vi "Init.vi"(10 "String Indicator":string) -> (3 "String Indicator Msg Strategy out":refnum<class "String Indicator Msg Strategy.lvclass">)   [LabVIEW 2021, in "jettl Msg String Indicator.lvlib" / "String Indicator Msg Strategy.lvclass"]
uses:
  String Indicator Msg Strategy.lvclass
  String Indicator Msg Strategy.lvclass/String Indicator Msg Strategy.ctl
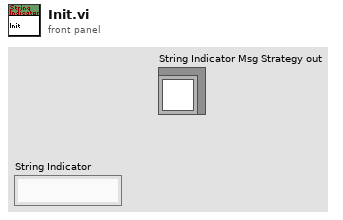
[diagram p1: front panel]
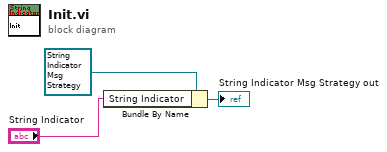
[diagram p0: block diagram]
diagram:
  n1 = Bundle By Name(cluster=refnum<class "String Indicator Msg Strategy.lvclass"> refnum ("String Indicator Ref.lvlib:String Indicator Msg.lvclass"), "String Indicator"="String Indicator") -> (→"String Indicator Msg Strategy out":refnum<class "String Indicator Msg Strategy.lvclass">)
